vi "sequ2.vi"   [LabVIEW 2019]
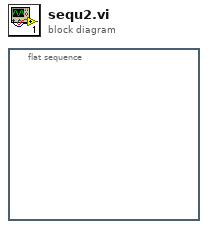
[diagram p0: block diagram]
diagram:
  n1 = flat-sequence {
    frame #0 {
    }
  }
